vi "自定义双按钮对话框.vi"(8 "取消文本":string, 9 "确定文本":string, 11 "消息":string) -> (2 "正式版/测试版输出":bool, 3 "输出":bool)   [LabVIEW 2016, in "数据传输系统-02.lvlib"]
panel:
  in  "正式版/测试版":bool
  in  "取消":bool
  out "计时":i32
  in  "确定":bool
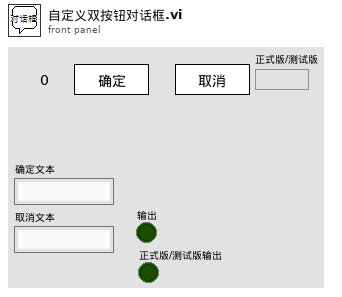
[diagram p1: front panel]
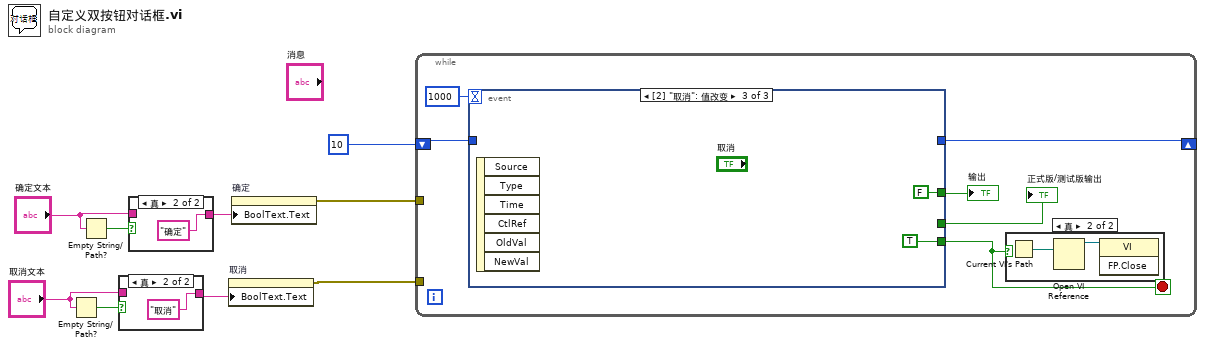
[diagram p0: block diagram]
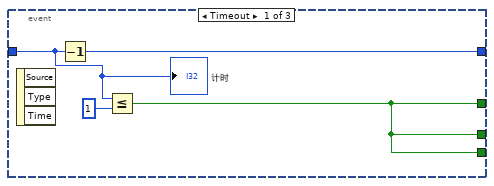
[diagram p3: hidden frame]
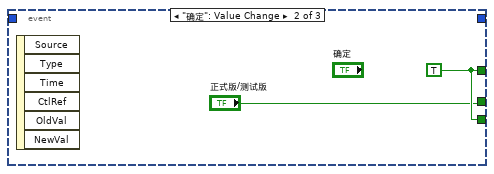
[diagram p4: hidden frame]
diagram:
  n1 = Empty String/Path?(string/path="取消文本") -> (empty?=w4:bool)
  n2 = Empty String/Path?(string/path="确定文本") -> (empty?=w7:bool)
  n3 = case shown="真" w4 {
    tunnel: [w10 "取消"] -> w2
    tunnel: "取消文本" -> [w10 _]
    frame False {
    }
    frame True {
    }
  }
  n4 = case shown="真" w7 {
    tunnel: [w12 "确定"] -> w6
    tunnel: "确定文本" -> [w12 _]
    frame False {
    }
    frame True {
    }
  }
  n5 = property on="取消" class="Bool"("BoolText.Text"=w2) -> (error out=w1:errorcluster)  [unwired: 2 in, 1 out]
  n6 = property on="确定" class="Bool"("BoolText.Text"=w6) -> (error out=w8:errorcluster)  [unwired: 2 in, 1 out]
  n7 = while {
    shift-right: [w19] -> _
    shift-left: 10 -> [w18]
    tunnel: w8 -> [_]
    tunnel: w1 -> [_]
    stop <- w15 stop-if-true
    n8 = event shown="[2] \"取消\": 值改变" {
      selector: _ -> [_ _ _]
      dyn-events: _ -> [_ _ _]
      timeout: 1000 -> [_ _ _]
      tunnel: [w25 _ _] -> w19
      tunnel: w18 -> [w24 _ _]
      tunnel: [w22 w27 FALSE ("确定")] -> w16
      tunnel: [w22 w27 TRUE] -> w15
      tunnel: [w22 "正式版/测试版" _] -> w14
      event Timeout {
        n9 = event-data() -> ()  [unwired: 1 in, 3 out]
        n10 = Decrement(x=w24) -> (x-1=w25:i32)
        n11 = Less Or Equal?(x=w24, y=1) -> (x <= y?=w22:bool)
        "计时" <- w24
      }
      event "确定": Value Change {
        w27 = TRUE ("确定")
        n12 = event-data() -> ()  [unwired: 1 in, 6 out]
      }
      event "取消": Value Change {
        n13 = event-data() -> ()  [unwired: 1 in, 6 out]
      }
    }
    "输出" <- w16
    "正式版/测试版输出" <- w14
    n14 = case shown="真" w15 {
      frame False {
      }
      frame True {
        n15 = Current VI's Path() -> (path=w21:path)
        n16 = Open VI Reference(vi path=w21) -> (vi reference=w20:refnum<vi>)  [unwired: 5 in, 1 out]
        n17 = invoke class="VI" method="FP.Close"(reference=w20) -> ()  [unwired: 2 in, 3 out]
      }
    }
  }
